vi "Open File.vi"(8 "error in (no error)":errorcluster, 11 "Spectrum Recorder in":refnum<class "Spectrum Recorder too.lvclass">) -> (0 "error out":errorcluster, 3 "Spectrum Recorder out":refnum<class "Spectrum Recorder too.lvclass">)   [LabVIEW 2019, in "Spectrum Recorder too.lvclass"]
uses:
  Spectrum Recorder too.lvclass
  C:/GitHub/LabActor/Template Module/Template Module.lvclass
  C:/Program Files/National Instruments/LabVIEW 2019/vi.lib/ActorFramework/Actor/Actor.lvclass
  Plots/Plot types.ctl
  NHMFL_Core/Libraries/Red Pitaya/RP Core/Red Pitaya Transceiver Driver/Internal Spectrum Configuration.ctl
  Spectrum Recorder too.lvclass/Spectrum Recorder too.ctl
  Template Module/Template Module.lvclass/Template Module.ctl
  <vilib>/ActorFramework/Actor/Actor.lvclass/Actor.ctl
  Controllers/Application Controller Messages/New Data File Msg/New Data File Msg.lvclass/New Data File Msg.ctl
  <vilib>/ActorFramework/Message Enqueuer/Message Enqueuer.lvclass/Message Enqueuer.ctl
  Template Module/Read Name.vi
  Read Fine region centers.vi
  Template Module/Read Logger.vi
  Template Module/Write Logger.vi
  <vilib>/ActorFramework/Message Enqueuer/Enqueue.vi
  Controllers/Application Controller Messages/New Data File Msg/New Data File Msg.lvclass
  C:/Program Files/National Instruments/LabVIEW 2019/vi.lib/ActorFramework/Message/Message.lvclass
  Read Spectrum Recorder Configuration.vi
  <vilib>/ActorFramework/Message Priority Queue/Priority Enqueue.vi
  Loggers/Logger/Logger.lvclass
  <vilib>/ActorFramework/Actor/Actor.lvclass
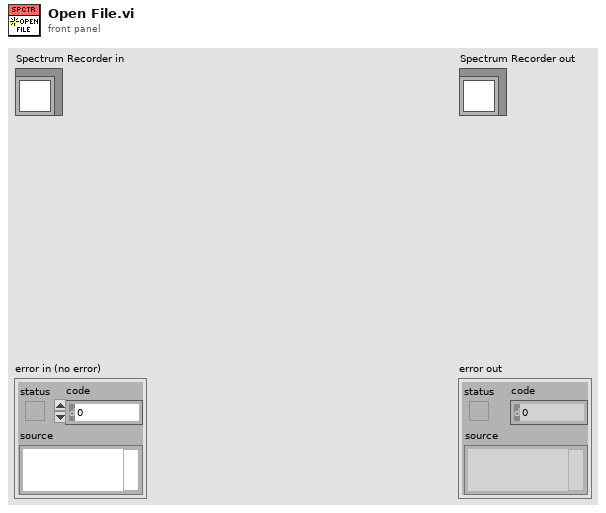
[diagram p1: front panel]
types:
  T1 = typedef "Plot types.ctl" = enum16{"Waveform Plot", "XY Plot", "Full XY"}
  T2 = typedef "Internal Spectrum Configuration.ctl" = cluster{"Start frequency":dbl, "End frequency":dbl, "Coarse step":dbl, "Step duration":dbl, "Red Pitaya address":string, "Open plot \non start":bool, "Fine region centers":dbl[], "Regions width":dbl, "Fine step":dbl, "Pause between scans":dbl, "Clear rgs on start":bool, "Output amplitude":dbl}
  T3 = typedef "Spectrum Configuration.ctl" = cluster{"Start frequency":dbl, "End frequency":dbl, "Coarse step":dbl, "Step duration":dbl, "Red Pitaya address":string, "Open plot \non start":bool, "Regions width":dbl, "Fine step":dbl, "Pause between scans":dbl, "Clear rgs on start":bool, "Output amplitude":dbl, "Append measurements":string[]}
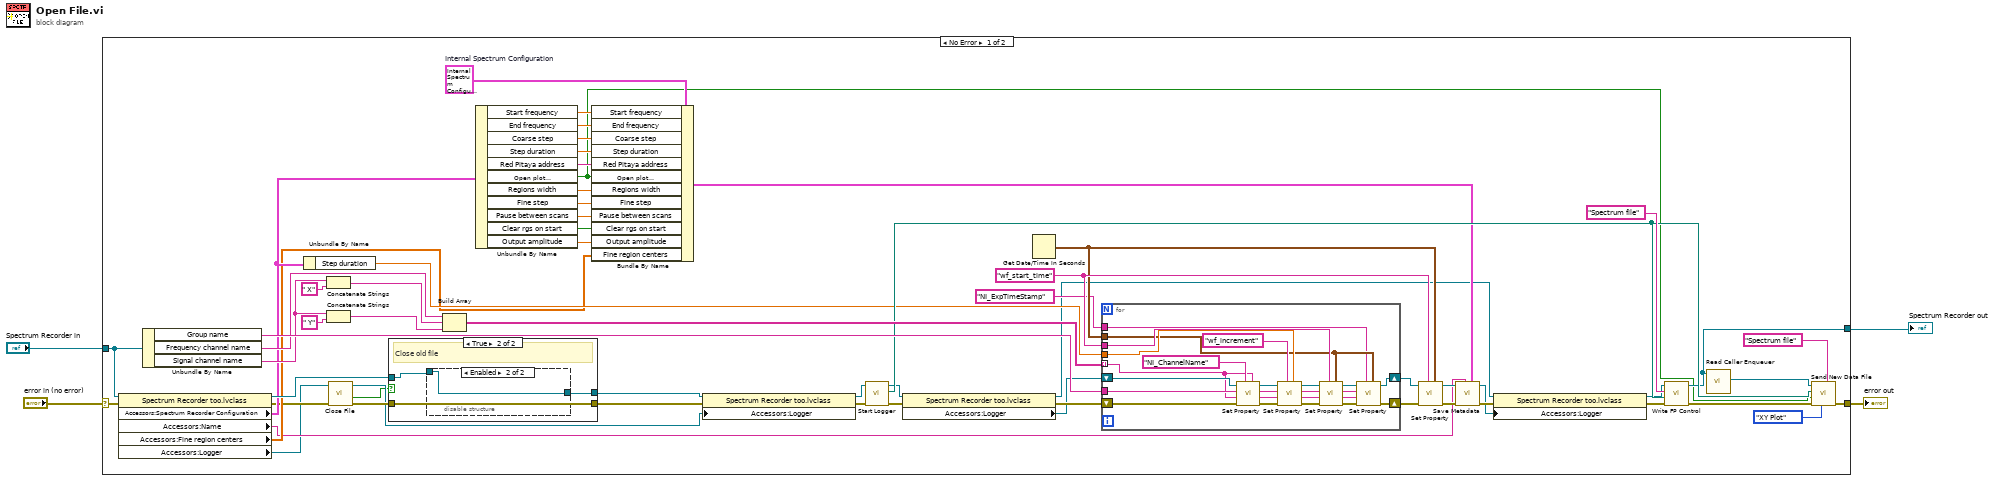
[diagram p0: block diagram]
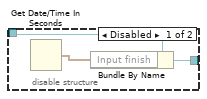
[diagram p3: hidden frame]
diagram:
  n1 = case shown="No Error" "error in (no error)" {
    selector: "error in (no error)" -> [w63 w100]
    tunnel: [w49 w100] -> w3
    tunnel: [w46 w99] -> w1
    tunnel: "Spectrum Recorder in" -> [w62 w99]
    frame No Error {
      w35 = T2 {"Start frequency"=500000.0, "End frequency"=2000000.0, "Coarse step"=100.0, "Step duration"=0.004, "Red Pitaya address"="192.168.1.100", "Open plot \non start"=FALSE, "Fine region centers"=[], "Regions width"=2000.0, "Fine step"=1.0, "Pause between scans"=0.0, "Clear rgs on start"=FALSE, "Output amplitude"=1.0}  # Internal Spectrum Configuration
      w38 = "wf_start_time"
      n2 = property class="Spectrum Recorder too.lvclass"(reference=w62, error in=w63) -> (reference out=w59:refnum<class "Spectrum Recorder too.lvclass">, error out=w12:errorcluster, "Accessors:Spectrum Recorder Configuration"=w34:T3, "Accessors:Name"=w18:string, "Accessors:Fine region centers"=w23:dbl[], "Accessors:Logger"=w10:refnum<class "Logger.lvclass">)
      n3 = Unbundle By Name(w62) -> ("Group name"=w65:string, "Frequency channel name"=w64:string, "Signal channel name"=w54:string)
      n4 = Unbundle By Name(w34) -> ("Step duration"=w43:dbl)
      n5 = Concatenate Strings(w54, " X" ("string")) -> (w55:string)
      n6 = Concatenate Strings(w54, " Y" ("string")) -> (w53:string)
      n7 = call-dynamic "Close File.vi"("error in (no error)"=w12, "Logger in"=w10) -> ("error out"=w11:errorcluster, "Actually closed"=w5:bool, "Logger out"=w6:refnum<class "Logger.lvclass">)  [unwired: 6 in, 1 out]
      n8 = case shown="True" w5 {
        tunnel: w11 -> [w91 w92]
        tunnel: [w91 w92] -> w60
        tunnel: w59 -> [w90 w94]
        tunnel: [w90 w93] -> w8
        frame False {
        }
        frame True {
          # "Close old file"
          n9 = disable-structure shown="Enabled" {
            disable-tunnel: w94 -> [w97 w98]
            disable-tunnel: [w96 w98] -> w93
            frame Disabled {
              n10 = Get Date/Time In Seconds() -> (seconds since 1Jan1904=w95:timestamp)
              n11 = Bundle By Name(cluster=w97, "Input finish"=w95) -> (w96:refnum<class "Spectrum Recorder too.lvclass">)
            }
            frame Enabled {
            }
          }
        }
      }
      n12 = Build Array(w64, w55, w53) -> (w61:string[])
      n13 = Unbundle By Name(w34) -> ("Start frequency"=w33:dbl, "End frequency"=w32:dbl, "Coarse step"=w31:dbl, "Step duration"=w30:dbl, "Red Pitaya address"=w29:string, "Open plot \non start"=w13:bool, "Regions width"=w28:dbl, "Fine step"=w27:dbl, "Pause between scans"=w26:dbl, "Clear rgs on start"=w25:bool, "Output amplitude"=w24:dbl)
      n14 = Bundle By Name(cluster=w35, "Start frequency"=w33, "End frequency"=w32, "Coarse step"=w31, "Step duration"=w30, "Red Pitaya address"=w29, "Open plot \non start"=w13, "Regions width"=w28, "Fine step"=w27, "Pause between scans"=w26, "Clear rgs on start"=w25, "Output amplitude"=w24, "Fine region centers"=w23) -> (w22:T2)
      n15 = property class="Spectrum Recorder too.lvclass"(reference=w8, error in=w60, "Accessors:Logger"=w6) -> (reference out=w7:refnum<class "Spectrum Recorder too.lvclass">, error out=w9:errorcluster)
      n16 = call-dynamic "Start Logger.vi"("error in (no error)"=w9, "Worker in"=w7) -> ("error out"=w58:errorcluster, "File Path"=w48:path, "Worker out"=w20:refnum<class "Spectrum Recorder too.lvclass">)  [unwired: 7 in]
      n17 = property class="Spectrum Recorder too.lvclass"(reference=w20, error in=w58) -> (reference out=w16:refnum<class "Spectrum Recorder too.lvclass">, error out=w21:errorcluster, "Accessors:Logger"=w19:refnum<class "Logger.lvclass">)
      n18 = Get Date/Time In Seconds() -> (seconds since 1Jan1904=w37:timestamp)
      n19 = for {
        tunnel: w65 -> [w88]
        tunnel: w61 -> [w85] mode=indexing
        shift-right: [w70] -> w40
        shift-left: w19 -> [w89]
        shift-right: [w71] -> w42
        shift-left: w21 -> [w87]
        tunnel: w43 -> [w75]
        tunnel: w37 -> [w69]
        tunnel: w38 -> [w74]
        tunnel: "NI_ExpTimeStamp" -> [w68]
        n20 = call-dynamic "Set Property.vi"("property value"=w85, "property name"="NI_ChannelName", "error in (no error)"=w87, "channel name"=w85, "group name"=w88, "Logger in"=w89) -> ("error out"=w84:errorcluster, "channel name out"=w79:string, "group name out"=w80:string, "Logger out"=w83:refnum<class "Logger.lvclass">)  [unwired: 2 in]
        n21 = call-dynamic "Set Property.vi"("property value"=w75, "property name"="wf_increment", "error in (no error)"=w84, "channel name"=w79, "group name"=w80, "Logger in"=w83) -> ("error out"=w81:errorcluster, "channel name out"=w78:string, "group name out"=w77:string, "Logger out"=w82:refnum<class "Logger.lvclass">)  [unwired: 2 in]
        n22 = call-dynamic "Set Property.vi"("property value"=w69, "property name"=w74, "error in (no error)"=w81, "channel name"=w78, "group name"=w77, "Logger in"=w82) -> ("error out"=w72:errorcluster, "channel name out"=w66:string, "group name out"=w67:string, "Logger out"=w73:refnum<class "Logger.lvclass">)  [unwired: 2 in]
        n23 = call-dynamic "Set Property.vi"("property value"=w69, "property name"=w68, "error in (no error)"=w72, "channel name"=w66, "group name"=w67, "Logger in"=w73) -> ("error out"=w71:errorcluster, "Logger out"=w70:refnum<class "Logger.lvclass">)  [unwired: 2 in, 2 out]
      }
      n24 = call-dynamic "Set Property.vi"("property value"=w37, "property name"=w38, "error in (no error)"=w42, "Logger in"=w40) -> ("error out"=w41:errorcluster, "Logger out"=w39:refnum<class "Logger.lvclass">)  [unwired: 4 in, 2 out]
      n25 = call-dynamic "Save Metadata.vi"("property value"=w22, "name"=w18, "error in (no error)"=w41, "Logger in"=w39) -> ("error out"=w52:errorcluster, "Logger out"=w15:refnum<class "Logger.lvclass">)  [unwired: 4 in, 2 out]
      n26 = property class="Spectrum Recorder too.lvclass"(reference=w16, error in=w52, "Accessors:Logger"=w15) -> (reference out=w14:refnum<class "Spectrum Recorder too.lvclass">, error out=w17:errorcluster)
      n27 = call-dynamic "Write FP Control.vi"("error in (no error)"=w17, "Control Value"=w48, "Control Name"="Spectrum file", "Measure Object in"=w14) -> ("error out"=w47:errorcluster, "Measure Object out"=w46:refnum<class "Spectrum Recorder too.lvclass">)  [unwired: 6 in]
      n28 = call <vilib>:"Read Caller Enqueuer.vi"("Actor"=w46) -> ("Caller Enqueuer"=w50:refnum<class "Message Enqueuer.lvclass">)  [unwired: 10 in]
      n29 = call "Send New Data File.vi"("Plot group"="Spectrum file", "Plot type"=Plot_types."XY Plot", "error in (no error)"=w47, "New plot if not open"=w13, "File"=w48, "Message Enqueuer"=w50) -> ("error out"=w49:errorcluster)  [unwired: 4 in, 1 out]
    }
    frame Error {
    }
  }
  "error out" <- w3
  "Spectrum Recorder out" <- w1
